vi "Read Working Values.vi"(7 "Unit Address (1)":u8=1, 8 "error in (no error)":errorcluster, 11 "VISA resource name":refnum<visa-resource-name>) -> (0 "error out":errorcluster, 1 "Working Output (0)":i32, 2 "Working Setpoint (0)":i32, 3 "VISA resource name out":refnum<visa-resource-name>)   [LabVIEW 2014, in "Eurotherm 35xx Series.lvlib"]
doc: "This VI returns Working Values."
uses:
  <instrlib>/Eurotherm 35xx Series/Eurotherm 35xx Series.lvlib
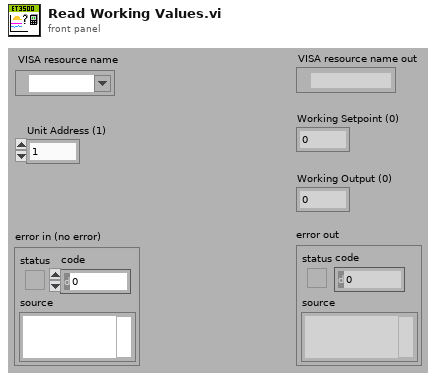
[diagram p1: front panel]
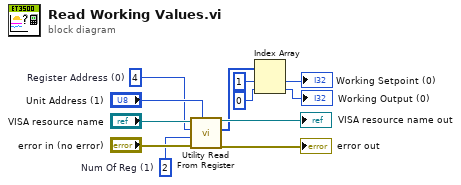
[diagram p0: block diagram]
diagram:
  w4 = 4  # Register Address (0)
  w7 = u16 2  # Num Of Reg (1)
  n1 = call <instrlib>:"Utility Read From Register.vi"("Unit Address (1)"="Unit Address (1)", "error in (no error)"="error in (no error)", "Num Of Reg (1)"=w7, "Register Address (0)"=w4, "VISA resource name"="VISA resource name") -> ("error out"=→"error out":errorcluster, "Data"=w6:i16[], "VISA resource name out"=→"VISA resource name out":refnum<visa-resource-name>)  [unwired: 4 in]
  n2 = Index Array(array=w6, index #1=1 ("index"), index #2=0 ("index")) -> (element #1=→"Working Setpoint (0)":i16, element #2=→"Working Output (0)":i16)
